vi "Read FunctionIniFilePath.vi"(8 "error in (no error)":errorcluster, 11 "Simulation in":refnum<class "Simulation.lvclass">) -> (0 "error out":errorcluster, 2 "FunctionIniFilePath":path, 3 "Simulation out":refnum<class "Simulation.lvclass">)   [LabVIEW 2018, in "DigitizerPlugins.lvlib" / "Simulation.lvclass"]
uses:
  Simulation.lvclass
  Simulation.lvclass/Simulation.ctl
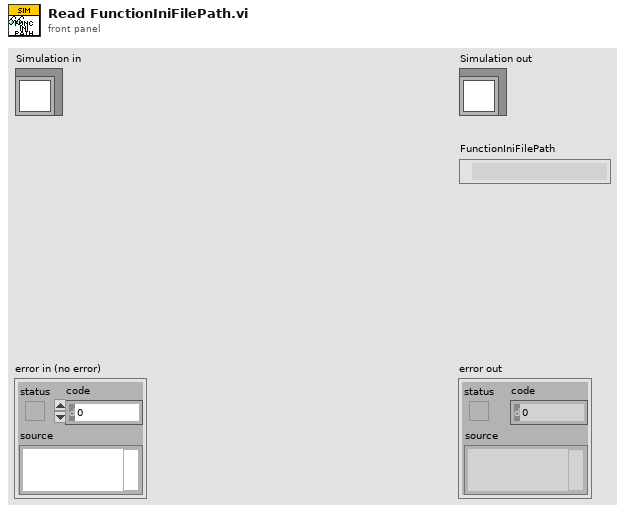
[diagram p1: front panel]
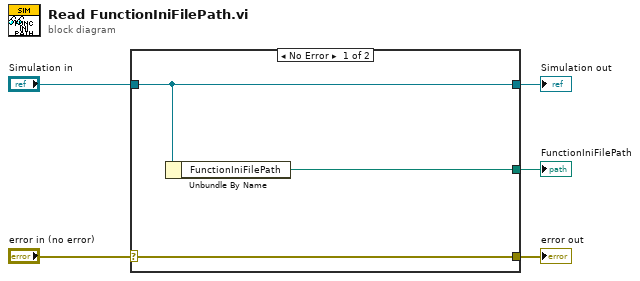
[diagram p0: block diagram]
diagram:
  n1 = case shown="No Error" "error in (no error)" {
    selector: "error in (no error)" -> [w8 w9]
    tunnel: [w8 w9] -> w4
    tunnel: [w7 w10] -> w2
    tunnel: "Simulation in" -> [w7 w10]
    tunnel: [w6 _] -> w1
    frame No Error {
      n2 = Unbundle By Name(w7) -> ("FunctionIniFilePath"=w6:path)
    }
    frame Error {
    }
  }
  "error out" <- w4
  "Simulation out" <- w2
  "FunctionIniFilePath" <- w1
